vi "Packet_encode_Int64.vi"(9 "Int64_Value":i64, 11 "RawData In":u8[](array[numeric])) -> (3 "RawData Out":u8[](array[numeric]))   [LabVIEW 2019, in "PhotonVisionLib.lvlib"]
doc: "Encode (or append) a 64 bit integer at the end of an array of bytes. No conversion is actually done, the memory is just copied to the end of the array.\n\nInputs\n - RawData In -- Array of bytes to be appended to..\n - In64_Value -- 64 bit integer the form of an INT 64 value.\n\nOutputs\n - RawData Out -- Array of bytes containing the appended value."
uses:
  PhotonVisionLib.lvlib
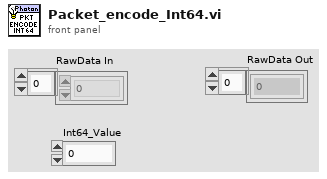
[diagram p1: front panel]
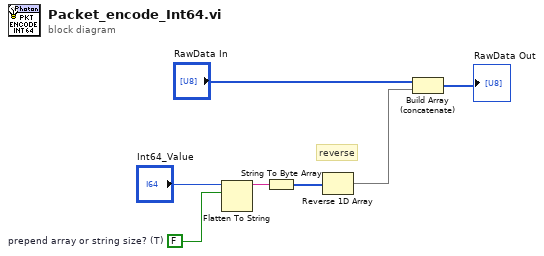
[diagram p0: block diagram]
diagram:
  w6 = FALSE  # prepend array or string size? (T)
  # "reverse"
  n1 = Flatten To String(anything="Int64_Value", prepend array or string size? (T)=w6) -> (data string=w4:string)  [unwired: 2 in, 2 out]
  n2 = String To Byte Array(string=w4) -> (unsigned byte array=w2:u8[])
  n3 = Reverse 1D Array(array=w2) -> (reversed array=w1:u8[])
  n4 = Build Array (concatenate)("RawData In", w1) -> (→"RawData Out":u8[])
